vi "SetIntValue.vi"(1 "error in (no error)":errorcluster, 2 "Int Value":i32, 3 "Feature Name":string, 4 "IGxDevice":refnum<k24>) -> (0 "error out":errorcluster)   [LabVIEW 2013, in "GxLVlib.lvlib"]
uses:
  GxLVlib.lvlib
  C:/Program Files/Daheng Imaging/GalaxySDK/Samples/LabVIEW SDK/x86/GxLVLib/dll/GxIAPINET.dll
  dll/GxIAPINET.dll
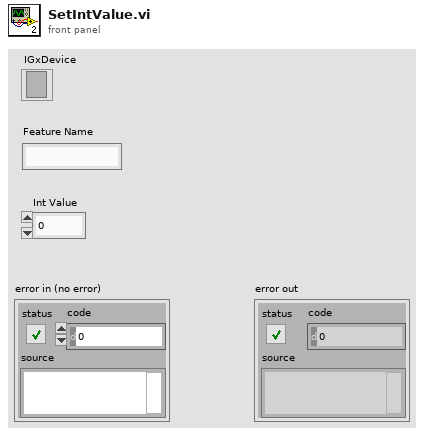
[diagram p1: front panel]
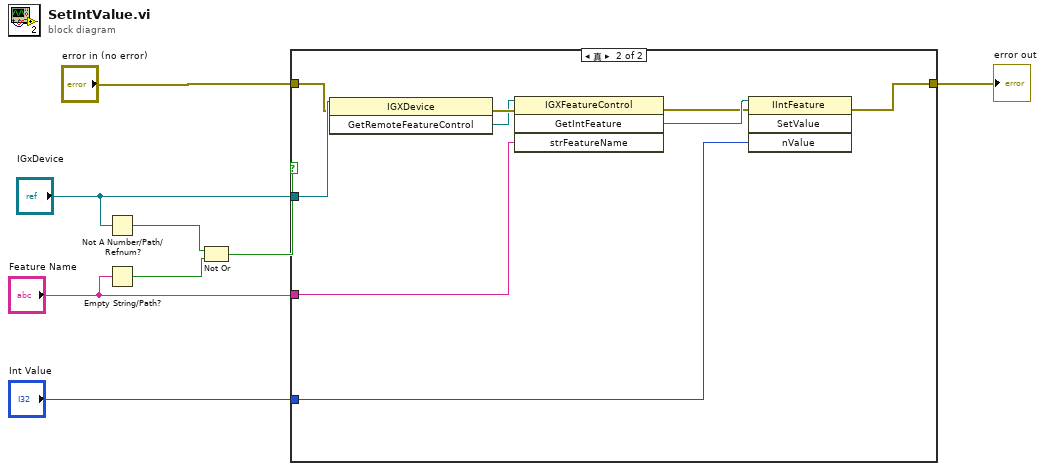
[diagram p0: block diagram]
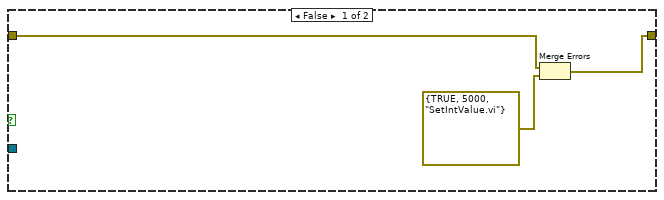
[diagram p2: hidden frame]
diagram:
  n1 = Not A Number/Path/Refnum?(number/path/refnum="IGxDevice") -> (NaN/Path/Refnum?=w8:bool)
  n2 = Empty String/Path?(string/path="Feature Name") -> (empty?=w7:bool)
  n3 = Not Or(1:w7, 2:w8) -> (0:w6:bool)
  n4 = case shown="真" w6 {
    tunnel: "error in (no error)" -> [w10 w15]
    tunnel: [w9 w14] -> w1
    tunnel: "IGxDevice" -> [_ w20]
    tunnel: "Feature Name" -> [_ w17]
    tunnel: "Int Value" -> [_ w16]
    frame False {
      n5 = Merge Errors(w10, errorcluster {TRUE, 5000, "SetIntValue.vi"}) -> (w9:errorcluster)
    }
    frame True {
      n6 = invoke class="IGXDevice" method="GetRemoteFeatureControl"(reference=w20, error in=w15) -> (error out=w19:errorcluster, "GetRemoteFeatureControl"=w18:refnum<k24>)  [unwired: 1 in, 1 out]
      n7 = invoke class="IGXFeatureControl" method="GetIntFeature"(reference=w18, error in=w19, "strFeatureName"=w17) -> (error out=w12:errorcluster, "GetIntFeature"=w13:refnum<k24>)  [unwired: 1 in, 2 out]
      n8 = invoke class="IIntFeature" method="SetValue"(reference=w13, error in=w12, "nValue"=w16) -> (error out=w14:errorcluster)  [unwired: 1 in, 3 out]
    }
  }
  "error out" <- w1
